vi "barometer.vi"(11 "Array in":dbl[](array[numeric])) -> (3 "Array out":dbl[](array[numeric]))   [LabVIEW 2017]
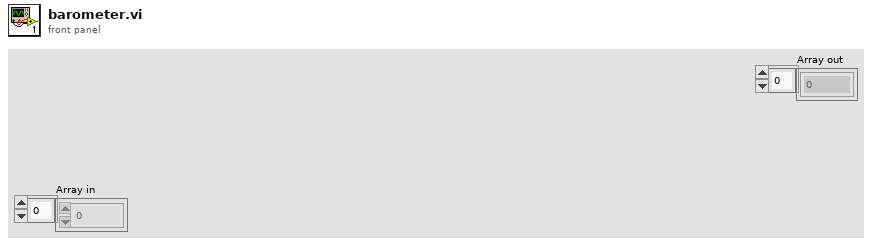
[diagram p1: front panel]
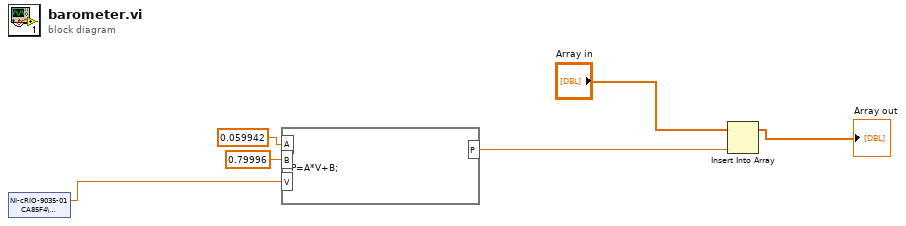
[diagram p0: block diagram]
diagram:
  n1 = shared-variable "NI-cRIO-9035-01CA85F4\\EtherCAT Master\\Device\\Mod1\\AI0"() -> (w1:dbl)  [unwired: 1 in, 1 out]
  n2 = formula code="P=A*V+B;"("V"=w1, "A"=0.059942 ("input variable"), "B"=0.79996 ("input variable")) -> ("P"=w6:dbl)
  n3 = Insert Into Array(array="Array in", new element=w6) -> (→"Array out":dbl[])  [unwired: 1 in]
